vi "Untitled 2.vi"() -> ()   [LabVIEW 2019]
uses:
  func.dll
panel:
  out "range":i32
  out "duration":i32
  out "f1":i32
  out "f0":i32
  out "array_length":i32
  out "type":i32
  out "array_pow":i32[](array[numeric])
  out "array_indice 2":i32[](array[numeric])
  in  "array_indice":i32[](array[numeric])
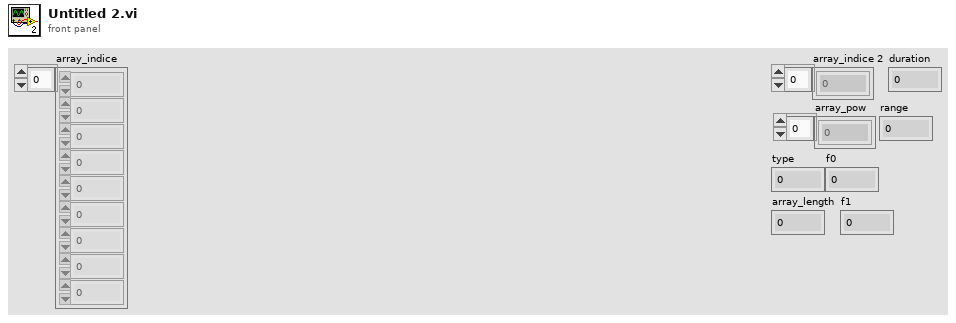
[diagram p1: front panel]
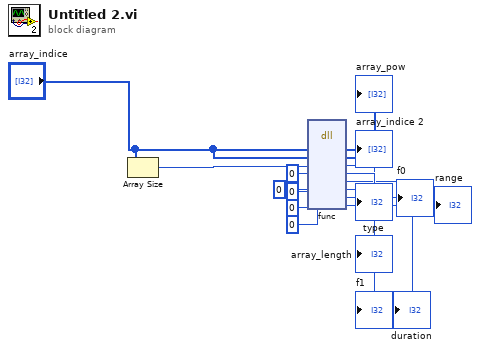
[diagram p0: block diagram]
diagram:
  n1 = Array Size(array="array_indice") -> (size(s)=w14:i32)
  n2 = dll-call lib="C:/Users/bilge/Documents/func/func.dll" fn="func"("array_indice"="array_indice", "array_pow"="array_indice", "array_length"=w14, "type"=0, "f0"=0, "f1"=0, "duration"=0, "range"=0) -> ("array_indice"=→"array_indice 2":i32[], "array_pow"=→"array_pow":i32[], "array_length"=→"array_length":i32, "type"=→"type":i32, "f0"=→"f0":i32, "f1"=→"f1":i32, "duration"=→"duration":i32, "range"=→"range":i32)  [unwired: 4 in, 2 out]
